vi "move axe.vi"(9 "Axe":dbl, 10 "Speed":dbl, 11 "Angle":dbl) -> ()   [LabVIEW 2017]
uses:
  Settings/Traverse-Settings-Global.vi
  ICNC/ICNC2.lvlib
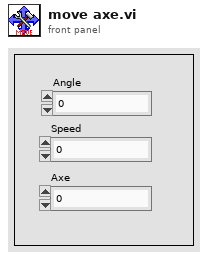
[diagram p1: front panel]
types:
  T1 = typedef "Settings-Control.ctl" = cluster{"Acceleration":dbl[], "Deceleration":dbl[], "Max Velocity":dbl[], "Speed":dbl, "Pulse/Degree":dbl, "Degre Factor":dbl[], "mm/rotation":dbl[], "Traverse Name":string}
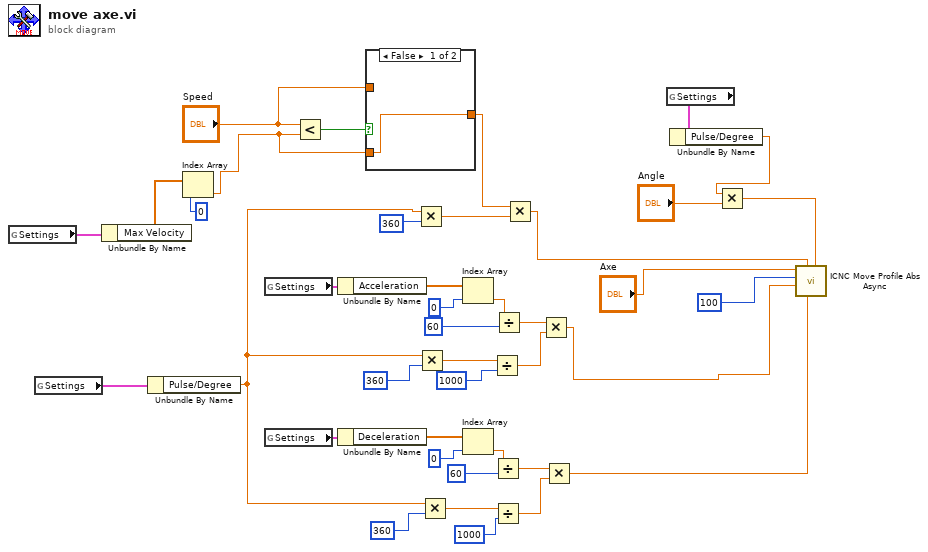
[diagram p0: block diagram]
diagram:
  n1 = global read "Traverse-Settings-Global.vi" "Settings"() -> (w3:T1)
  n2 = global read "Traverse-Settings-Global.vi" "Settings"() -> (w7:T1)
  n3 = Unbundle By Name(w3) -> ("Max Velocity"=w17:dbl[])
  n4 = Unbundle By Name(w7) -> ("Pulse/Degree"=w6:dbl)
  n5 = Index Array(array=w17, index=0) -> (element=w16:dbl)
  n6 = global read "Traverse-Settings-Global.vi" "Settings"() -> (w15:T1)
  n7 = global read "Traverse-Settings-Global.vi" "Settings"() -> (w11:T1)
  n8 = Less?(x="Speed", y=w16) -> (x < y?=w28:bool)
  n9 = Unbundle By Name(w15) -> ("Acceleration"=w14:dbl[])
  n10 = Unbundle By Name(w11) -> ("Deceleration"=w10:dbl[])
  n11 = case shown="False" w28 {
    tunnel: "Speed" -> [_ w42]
    tunnel: w16 -> [w41 _]
    tunnel: [w41 w42] -> w23
    frame False {
    }
    frame True {
    }
  }
  n12 = Multiply(x=w6, y=360) -> (x*y=w24:dbl)
  n13 = Multiply(x=w6, y=360) -> (x*y=w26:dbl)
  n14 = Multiply(x=w6, y=360) -> (x*y=w25:dbl)
  n15 = Index Array(array=w14, index=0) -> (element=w12:dbl)
  n16 = Index Array(array=w10, index=0) -> (element=w8:dbl)
  n17 = Divide(x=w26, y=1000) -> (x/y=w40:dbl)
  n18 = Divide(x=w8, y=60) -> (x/y=w36:dbl)
  n19 = Divide(x=w25, y=1000) -> (x/y=w35:dbl)
  n20 = Divide(x=w12, y=60) -> (x/y=w30:dbl)
  n21 = Multiply(x=w23, y=w24) -> (x*y=w1:dbl)
  n22 = Multiply(x=w30, y=w40) -> (x*y=w2:dbl)
  n23 = Multiply(x=w36, y=w35) -> (x*y=w21:dbl)
  n24 = global read "Traverse-Settings-Global.vi" "Settings"() -> (w5:T1)
  n25 = Unbundle By Name(w5) -> ("Pulse/Degree"=w4:dbl)
  n26 = Multiply(x=w4, y="Angle") -> (x*y=w19:dbl)
  n27 = call "ICNC Move Profile Abs Async.vi"("Position"=w19, "Decel"=w21, "Speed"=w1, "Accel"=w2, "FStartStop"=100, "Axe"="Axe") -> ()  [unwired: 4 in, 2 out]
